vi "MT_write.vi"(8 "error in":errorcluster, 9 "sampling rate":dbl, 10 "duration":dbl, 11 "data":dbl[][](array[numeric]) format="%0.2f") -> (0 "error out":errorcluster)   [LabVIEW 2019]
uses:
  <vilib>/DAQmx/write.llb/DAQmx Write (Analog 2D DBL NChan NSamp).vi
  <vilib>/DAQmx/create/channels.llb/DAQmx Create Channel (AO-Voltage-Basic).vi
  <vilib>/DAQmx/configure/timing.llb/DAQmx Timing (Sample Clock).vi
  <vilib>/DAQmx/miscellaneous.llb/DAQmx Fill In Error Info.vi
panel:
  in  "stop":bool
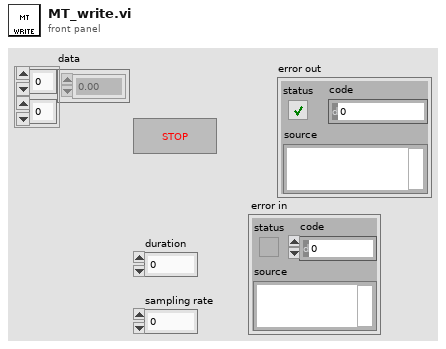
[diagram p1: front panel]
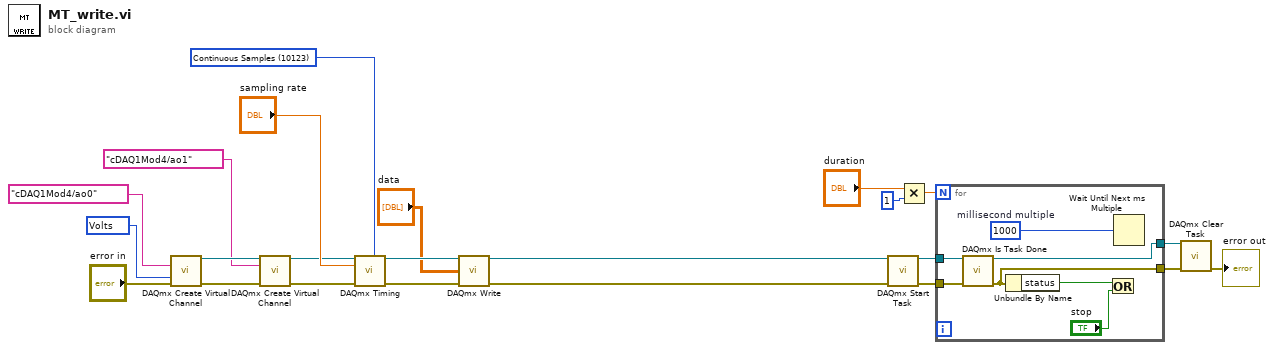
[diagram p0: block diagram]
diagram:
  w8 = 10348 items=["Volts"=10348, "From Custom Scale"=10065] ("units")
  w12 = 10123 items=["Finite Samples"=10178, "Continuous Samples"=10123] ("sample mode")
  n1 = call-poly <vilib>:"DAQmx Create Virtual Channel.vi"("physical channels"=tag "cDAQ1Mod4/ao0", "units"=w8, "error in"="error in") -> ("task out"=w6:refnum<k21>, "error out"=w5:errorcluster)  [unwired: 6 in, 5 out]
  n2 = call-poly <vilib>:"DAQmx Create Virtual Channel.vi"("task in"=w6, "physical channels"=tag "cDAQ1Mod4/ao1", "error in"=w5) -> ("task out"=w4:refnum<k21>, "error out"=w3:errorcluster)  [unwired: 11 in]
  n3 = call-poly <vilib>:"DAQmx Timing.vi"("task/channels in"=w4, "sample mode"=w12, "rate"="sampling rate", "error in"=w3) -> ("task out"=w18:refnum<k21>, "error out"=w19:errorcluster)  [unwired: 3 in, 7 out]
  n4 = call-poly <vilib>:"DAQmx Write.vi"("task/channels in"=w18, "data"="data", "error in"=w19) -> ("task out"=w13:refnum<k21>, "error out"=w14:errorcluster)  [unwired: 1 in, 10 out]
  n5 = call <vilib>:"DAQmx Start Task.vi"("task/channels in"=w13, "error in"=w14) -> ("task out"=w11:refnum<k21>, "error out"=w15:errorcluster)  [unwired: 12 out]
  n6 = Multiply(x="duration", y=1) -> (x*y=w21:dbl)
  n7 = for {
    N: w21 -> [_]
    tunnel: w11 -> [w30]
    tunnel: [w29] -> w16
    tunnel: w15 -> [w28]
    tunnel: [w26] -> w17
    w24 = u32 1000  # millisecond multiple
    n8 = call <vilib>:"DAQmx Is Task Done.vi"("task/channels in"=w30, "error in"=w28) -> ("task out"=w29:refnum<k21>, "error out"=w26:errorcluster)  [unwired: 1 in, 11 out]
    n9 = Unbundle By Name(w26) -> ("status"=w27:bool)
    n10 = Or(x=w27, y="stop") -> ()  [unwired: 1 out]
    n11 = Wait Until Next ms Multiple(millisecond multiple=w24) -> ()  [unwired: 1 out]
  }
  n12 = call <vilib>:"DAQmx Clear Task.vi"("task in"=w16, "error in"=w17) -> ("error out"=→"error out":errorcluster)  [unwired: 13 out]
